vi "Format Page.vi"() -> ()   [LabVIEW 2020, in "3D Plot.lvclass"]
uses:
  <vilib>/Math Plots/3D Math Plots/3D Plot/3D Plot/3D Plot.lvclass
  <vilib>/Math Plots/3D Math Plots/3D Plot/3D Plot/Typedef/Format Property.ctl
  <vilib>/Math Plots/3D Math Plots/3D Plot/3D Plot/Typedef/Dialog State.ctl
  <vilib>/Math Plots/3D Math Plots/3D Plot/3D Plot/Typedef/Temp Scene State.ctl
  <vilib>/Math Plots/3D Math Plots/3D Plot/3D Plot/Typedef/Temp Scene Property Action.ctl
panel:
  out "Format Testing":string
  in  "Caption Texts":string[](array[string])=["Numeric Format Codes", "Absolute Time Format Codes\n(must be within %< >T)", "Relative Time Format Codes\n(must be within %< >t)"]
  in  "Item Names":string[][][](array[string])=[[["Floating point notation", "%f"], ["Scientific notation", "%e"], ["Engineering notation", "%^e"], ["Automatic notation", "%#_g"], ["SI notation", "%p"], ["Decimal", "%d"], ["Unsigned decimal", "%u"], ["Hexadecimal", "%x"], ["Octal", "%o"], ["Binary", "%b"], ["A single percent character", "%%"], ["", ""], ["", ""], ["", ""], ["", ""], ["", ""], ["", ""], ["", ""], ["", ""], ["", ""], ["", ""], ["", ""], ["", ""]], [["Absolute time container", "%< >T"], ["Abbreviated weekday name", "%a"], ["Weekday name", "%A"], ["Abbreviated month name", "%b"], ["Month name", "%B"], ["Default date and time", "%c"], ["Day of month (01-31)", "%d"], ["Hour (24-hour clock) (00-23)", "%H"], ["Hour (12-hour clock) (01-12)", "%I"], ["Day of year (001-366)", "%j"], ["Month number (01-12)", "%m"], ["Minute (00-59)", "%M"], ["AM or PM flag", "%p"], ["Seconds (00-59)", "%S"], ["Fractional seconds with <digit>\nprecision", "%<digit> u"], ["Week number (00-53) with\nSunday as the first day of week 1", "%U"], ["Weekday number (0-6)", "%w"], ["Week number (00-53) with\nMonday as the first day of week 1", "%W"], ["Locale date", "%x"], ["Locale time", "%X"], ["Year within century (00-99)", "%y"], ["Year including century", "%Y"], ["Time zone", "%Z"]], [["Relative time container", "%< >t"], ["Weeks", "%W"], ["Days", "%D"], ["Hours", "%H"], ["Minutes", "%M"], ["Seconds", "%S"], ["Fractional seconds with <digit>\nprecision", "%<digit>u"], ["A single percent character", "%%"], ["", ""], ["", ""], ["", ""], ["", ""], ["", ""], ["", ""], ["", ""], ["", ""], ["", ""], ["", ""], ["", ""], ["", ""], ["", ""], ["", ""], ["", ""]]]
  out "Advanced Tab":enum32{"Standard", "Advanced"}(tab)
  out "Time/Date Tab":enum32{"numeric", "time"}(tab) caption="Tab Control 3"
  in  "HLP_just/pad":i32(ring) items=["Pad with spaces on left", "Pad with spaces on right", "Pad with zeros on left"]
  in  "HLP_UseMinWidth":bool caption="Use minimum field width"
  in  "HLP_trailing zeros":bool caption="Hide trailing zeros"
  in  "HLP_exponent":bool caption="Exponent in multiples of 3"
  in  "Precision Type":u16(ring) caption="Precision type" items=["Digits of precision", "Significant digits"]
  in  "Digits":i32 min=0
  in  "HLP_Minimum field width":i32 caption="Minimum field width" min=0
  in  "HLP_year-new":T1(radio)
  in  "HLP_MDY 2-new":T1(radio)
  in  "HLP_HMS-new":enum32{"Radio Selection 1", "Radio Selection 2"}(radio)
  in  "HLP_Hour Type-new":enum32{"Radio Selection 1", "Radio Selection 2"}(radio)
  in  "HLP_Date Type":u16(ring)=1 caption="Date Type" items=["Custom date format", "System date format", "Date unused"]
  in  "HLP_Digits":i32 caption="Digits" min=0
  in  "HLP_Time Type":u16(ring)=1 caption="Time Type" items=["Custom time format", "System time format", "Time unused"]
  in  "Type":i32(listbox)
  in  "HLP_Revert":bool caption="Revert"
  in  "HLP_Format Code List Type":u16(ring) items=["Numeric format codes", "Relative time format codes", "Absolute time format codes"]
  out "HLP_Valid Fmt String":bool=TRUE caption="Valid"
  in  "HLP_insert format code":bool caption="Insert into Format String"
  in  "HLP_percent codes":i32(listbox) caption="Numeric Format Codes"
  in  "ODF_Format String":string caption="Format string"
  in  "HLP_AdvancedFmt2":enum32{"Default mode", "Advanced mode"}(radio)
  in  "Active Axis":u16(ring) caption="Active axis" items=["X Axis", "Y Axis", "Z Axis"]
  in  "Event Registration":refnum<event-registration>
  out "Format Property Out":T2
  in  "Format Property In":T2
  # "Format"
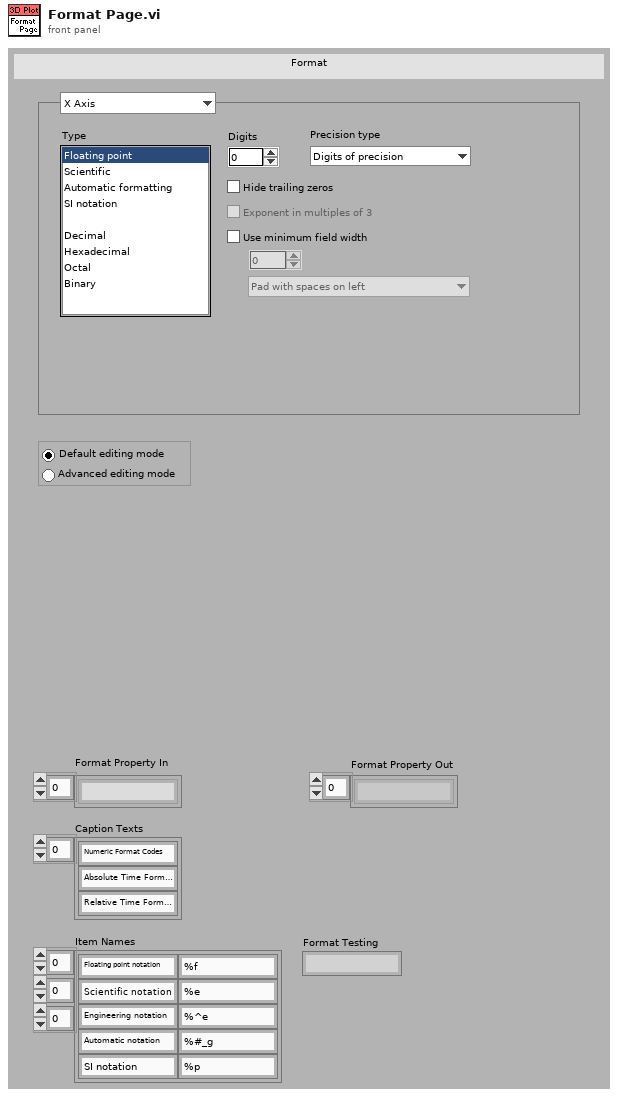
[diagram p1: front panel]
types:
  T1 = enum32{"Radio Selection 1", "Radio Selection 2", "Radio Selection 3"}
  T2 = typedef "3D Plot.lvclass/Format Property.ctl" = string[]
  T3 = typedef "3D Plot.lvclass/Dialog State.ctl" = enum16{"Initialize", "Read Porperty", "Write Property", "Idle", "Exit"}
  T4 = typedef "3D Plot.lvclass/Temp Scene Property Action.ctl" = enum16{"Graph Property", "Light Property", "Axis Property", "Value Pair Property", "Format Property", "Cursor Property", "Plot Specific Property"}
  T5 = typedef "3D Plot.lvclass/Temp Scene State.ctl" = enum16{"Create", "Update Scene", "Get Plot Representation", "Destory"}
  T6 = enum16{"number", "absolute time", "relative time"}
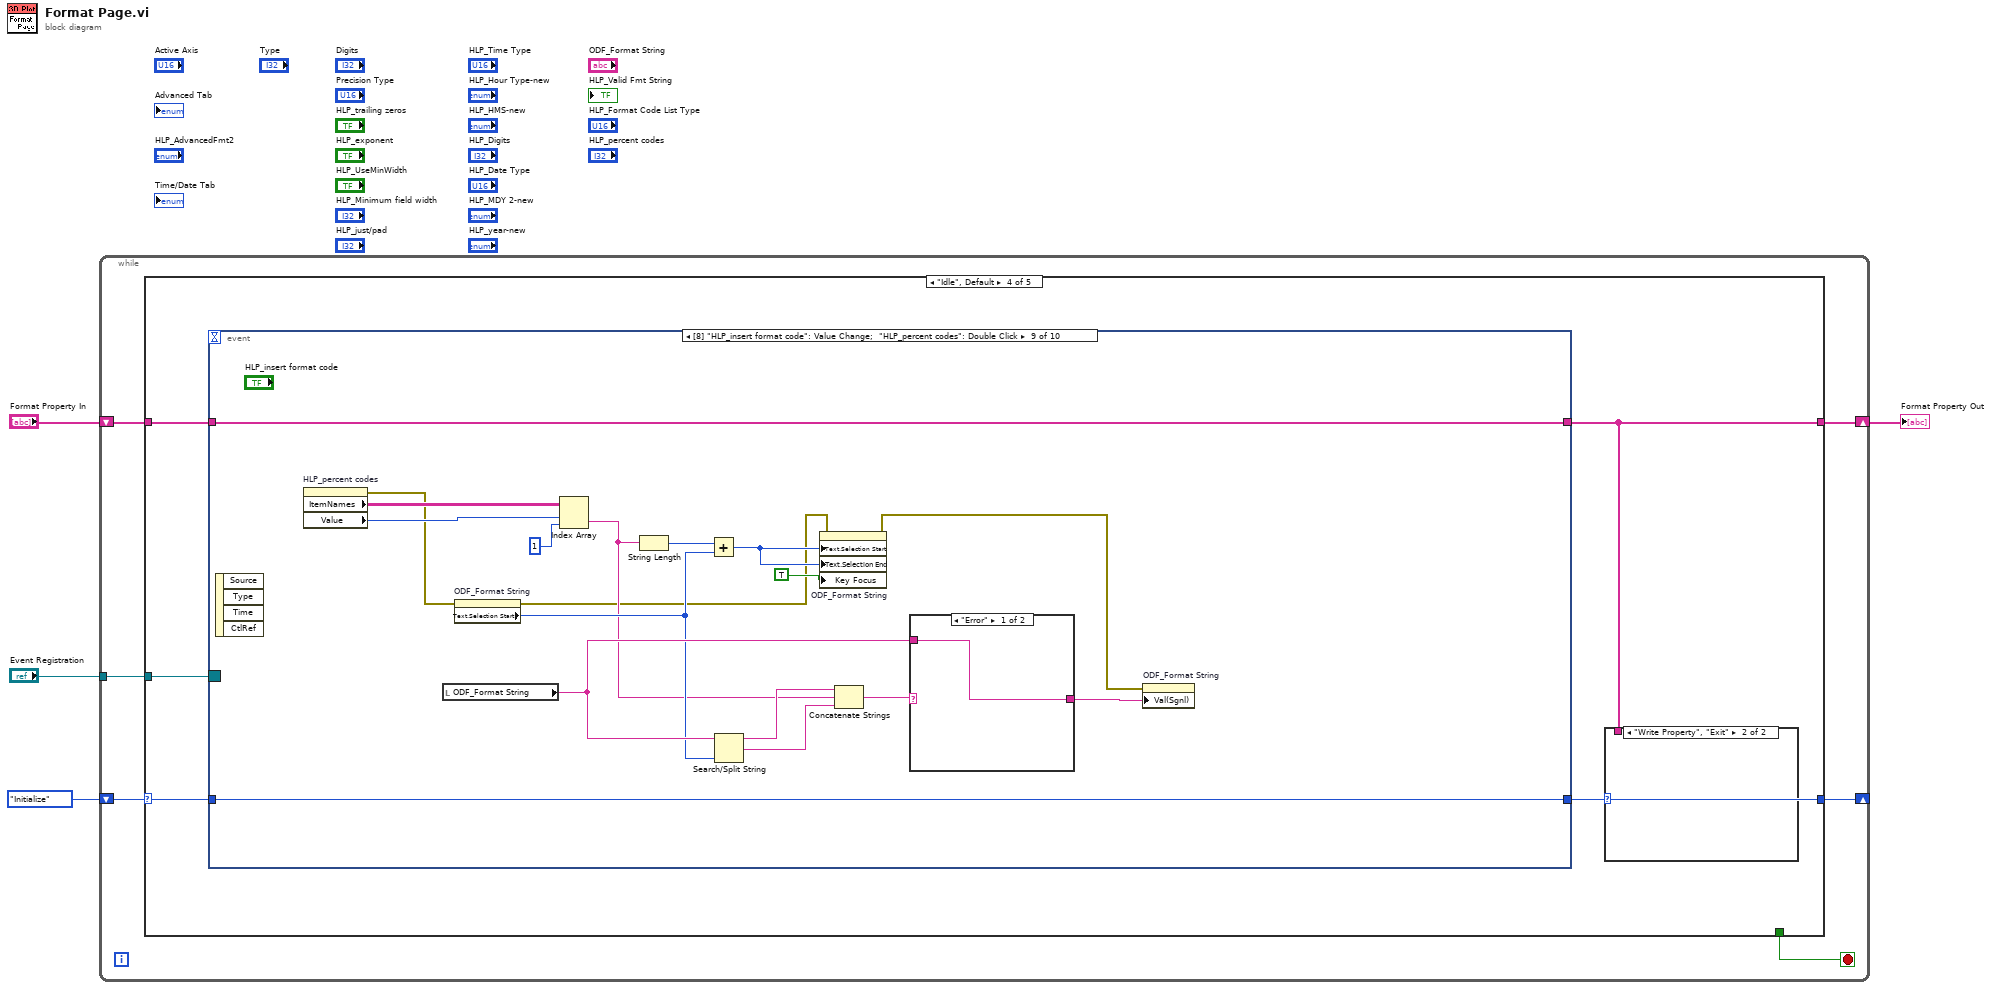
[diagram p0: block diagram]
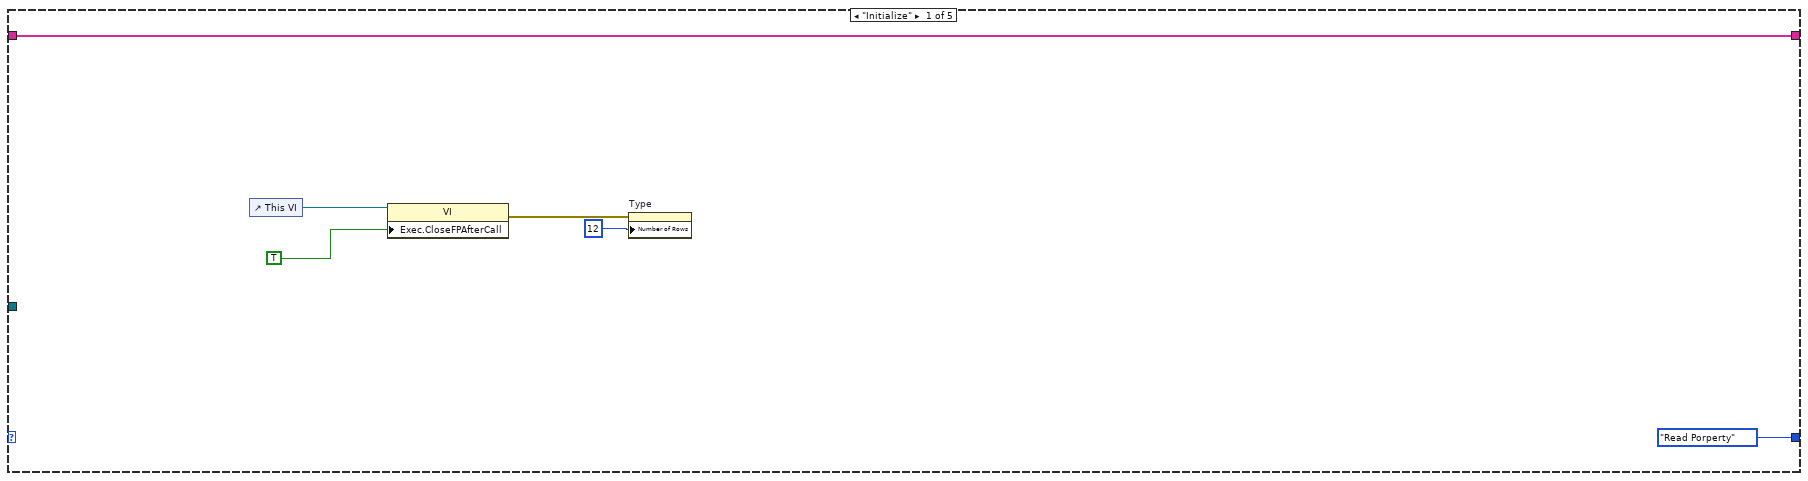
[diagram p2: hidden frame]
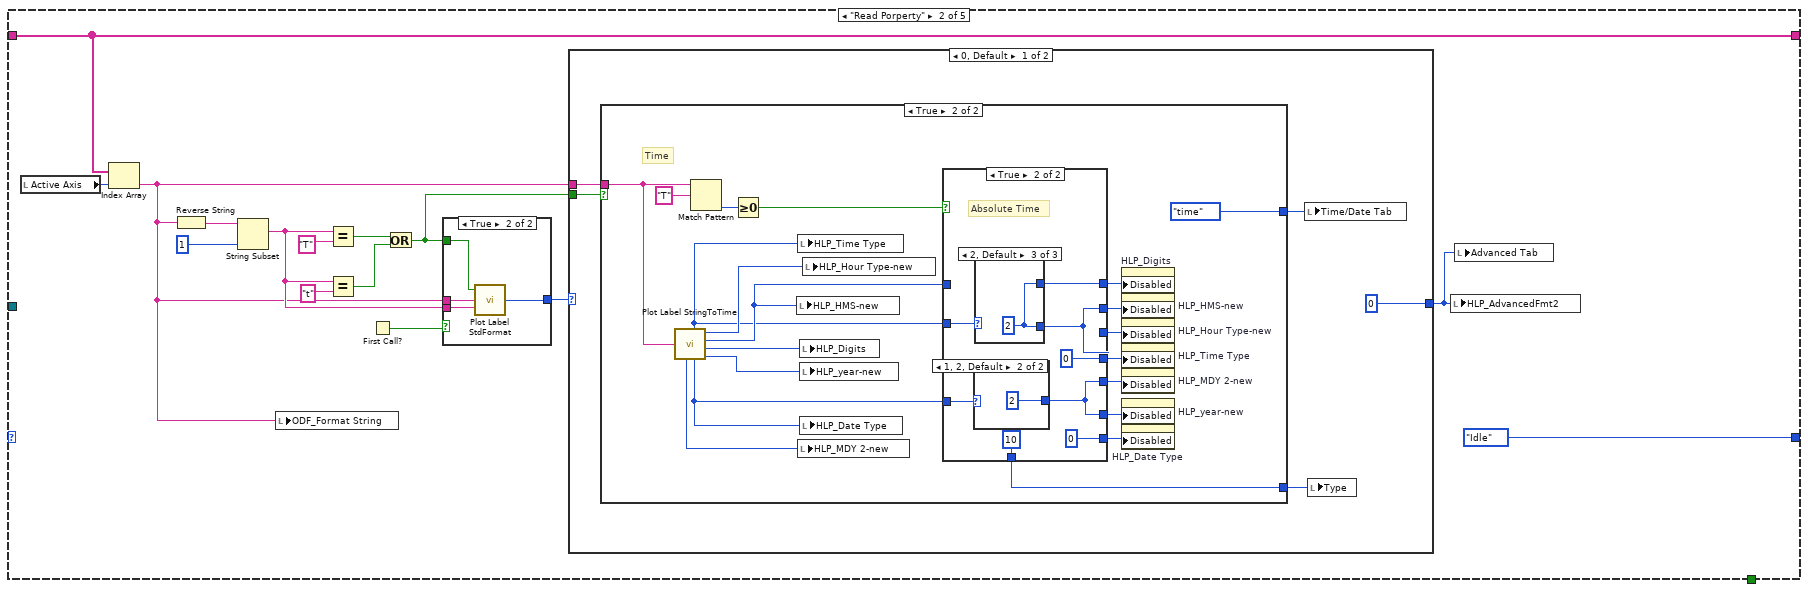
[diagram p3: hidden frame]
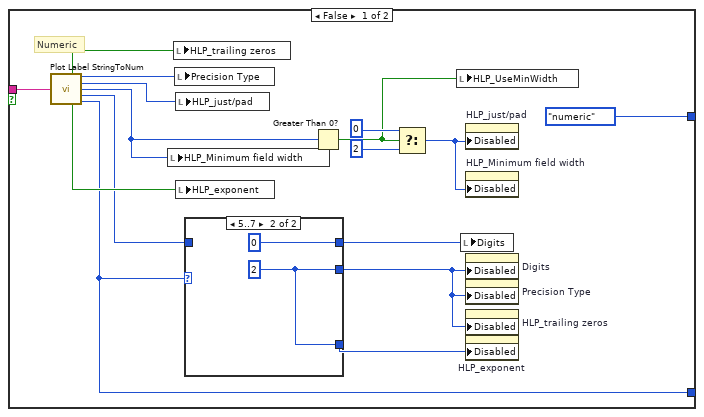
[diagram p4: hidden frame]
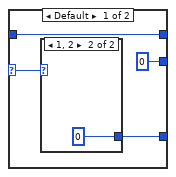
[diagram p5: hidden frame]
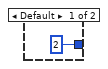
[diagram p6: hidden frame]
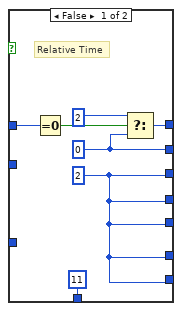
[diagram p7: hidden frame]
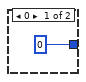
[diagram p8: hidden frame]
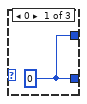
[diagram p9: hidden frame]
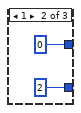
[diagram p10: hidden frame]
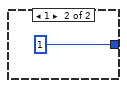
[diagram p11: hidden frame]
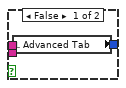
[diagram p12: hidden frame]
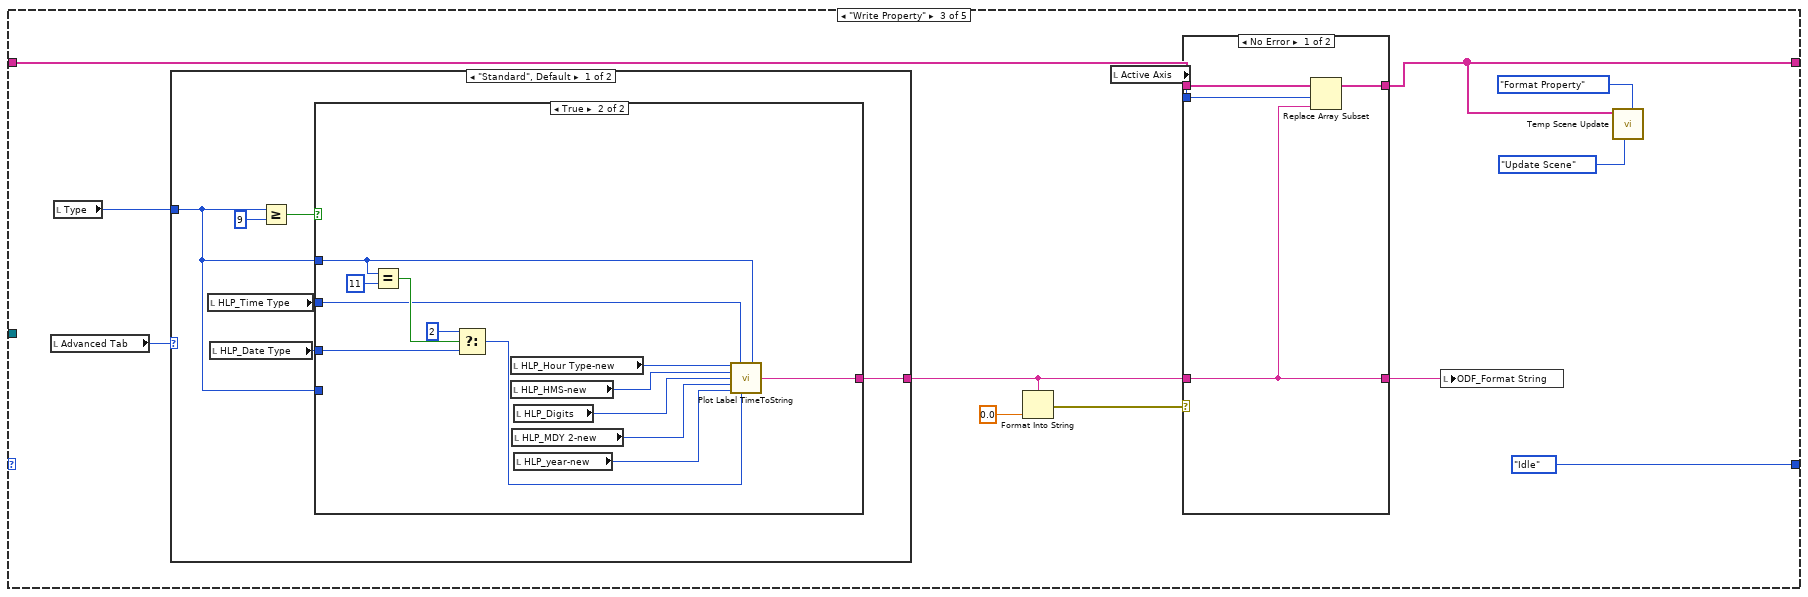
[diagram p13: hidden frame]
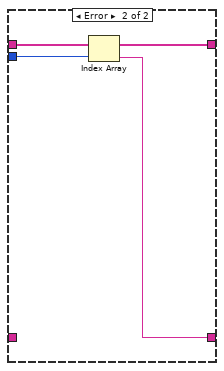
[diagram p14: hidden frame]
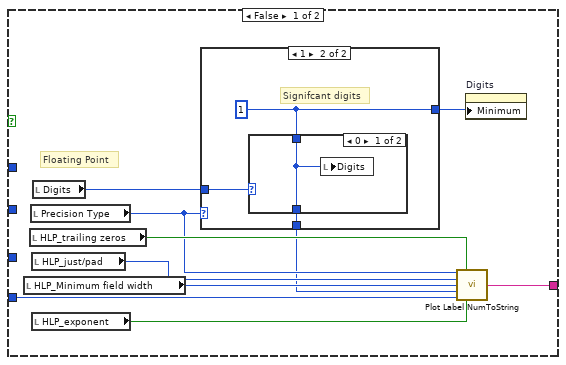
[diagram p15: hidden frame]
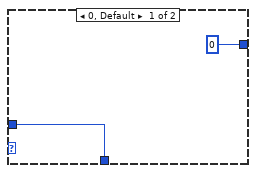
[diagram p16: hidden frame]
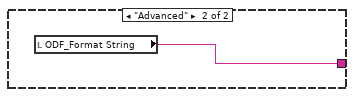
[diagram p18: hidden frame]
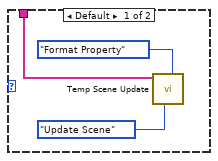
[diagram p19: hidden frame]
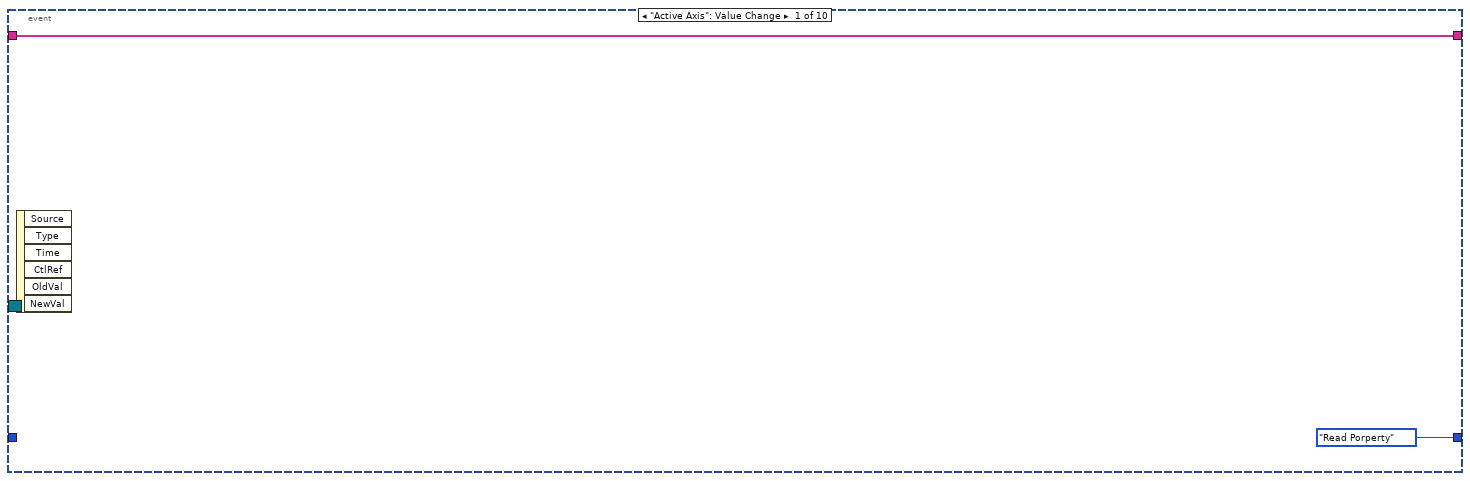
[diagram p20: hidden frame]
diagram:
  n1 = while {
    shift-right: [w5] -> w2
    shift-left: "Format Property In" -> [w10]
    shift-right: [w6] -> _
    shift-left: Dialog_State."Initialize" ("Enum") -> [w7]
    tunnel: "Event Registration" -> [w8]
    stop <- w9 stop-if-true
    n2 = case shown="\"Idle\", Default" w7 {
      selector: w7 -> [_ _ _ w166 _]
      tunnel: w10 -> [w16 w29 w114 w168 w387]
      tunnel: [w16 w29 w108 w165 w387] -> w5
      tunnel: [Dialog_State."Read Porperty" ("Enum") Dialog_State."Idle" Dialog_State."Idle" w164 Dialog_State."Exit"] -> w6
      tunnel: [_ _ _ _ TRUE] -> w9
      tunnel: w8 -> [_ _ _ w167 _]
      frame "Initialize" {
        n3 = control-ref of="This VI"() -> (w15:refnum<vi>)
        n4 = property class="VI"(reference=w15, "Exec.CloseFPAfterCall"=TRUE ("Execution:Close After Call")) -> (error out=w11:errorcluster)  [unwired: 1 in, 1 out]
        n5 = property on="Type" class="LstBox (strict)"(error in=w11, "Number of Rows"=u32 12) -> ()  [unwired: 1 in, 2 out]
      }
      frame "Read Porperty" {
        n6 = local read "Active Axis"() -> (w30:u16)
        n7 = Index Array(array=w29, index=w30) -> (element=w19:string)
        n8 = Reverse String(1:w19) -> (0:w24:string)
        n9 = String Subset(string=w24, length (rest)=1 ("length (rest)")) -> (substring=w28:string)  [unwired: 1 out]
        n10 = local write "ODF_Format String"(w19) -> ()
        n11 = Equal?(x=w28, y="T") -> (x = y?=w26:bool)
        n12 = Equal?(x=w28, y="t") -> (x = y?=w27:bool)
        n13 = First Call?() -> (First Call?: T/F=w21:bool)
        n14 = Or(x=w26, y=w27) -> (x .or. y?=w18:bool)
        n15 = case shown="True" w21 {
          tunnel: w28 -> [_ w105]
          tunnel: w18 -> [_ w107]
          tunnel: w19 -> [_ w106]
          tunnel: [w103 w104] -> w20
          frame False {
            n16 = local read "Advanced Tab"() -> (w103:enum32{"Standard", "Advanced"})
          }
          frame True {
            n17 = call <vilib>:"Plot Label StdFormat.vi"("Time Type"=w105, "Format String"=w106, "Type (false = numeric)"=w107) -> ("Custom"=w104:i32)
          }
        }
        n18 = case shown="0, Default" w20 {
          tunnel: w19 -> [w36 _]
          tunnel: w18 -> [w35 _]
          tunnel: [0 1] -> w17
          frame 0, Default {
            n19 = case shown="True" w35 {
              tunnel: w36 -> [w52 w78]
              tunnel: [w45 w69] -> w34
              tunnel: [enum32{"numeric", "time"}."numeric" ("Time/Date Tab") enum32{"numeric", "time"}."time" ("Time/Date Tab")] -> w33
              frame False {
                # "Numeric"
                n20 = call <vilib>:"Plot Label StringToNum.vi"("Format String"=w52) -> ("Hide trailing zeros"=w51:bool, "Digit Type"=w49:i32, "just/pad"=w48:i32, "Minimum Field Width"=w40:i32, "Digits of Precision"=w47:i32, "exponent"=w50:bool, "Numeric Format"=w45:i32)  [unwired: 8 out]
                n21 = local write "HLP_Minimum field width"(w40) -> ()
                n22 = local write "HLP_trailing zeros"(w51) -> ()
                n23 = local write "Precision Type"(w49) -> ()
                n24 = local write "HLP_just/pad"(w48) -> ()
                n25 = local write "HLP_exponent"(w50) -> ()
                n26 = case shown="5..7" w45 {
                  selector: w45 -> [w54 _]
                  tunnel: [u8 0 w59] -> w44
                  tunnel: w47 -> [w55 _]
                  tunnel: [w55 0 ("Digits of Precision")] -> w46
                  tunnel: [w53 w59] -> w43
                  frame Default {
                    n27 = case shown="1, 2" w54 {
                      tunnel: [u8 2 u8 0] -> w53
                      frame Default {
                      }
                      frame 1, 2 {
                      }
                    }
                  }
                  frame 5..7 {
                    w59 = u8 2
                  }
                }
                n28 = Greater Than 0?(x=w40) -> (x > 0?=w39:bool)
                n29 = Select(t=u8 0, s=w39, f=u8 2) -> (s? t:f=w38:u8)
                n30 = local write "HLP_UseMinWidth"(w39) -> ()
                n31 = local write "Digits"(w46) -> ()
                n32 = property on="HLP_just/pad" class="Ring (strict)"("Disabled"=w38) -> ()  [unwired: 2 in, 2 out]
                n33 = property on="HLP_Minimum field width" class="DigNum (strict)"("Disabled"=w38) -> ()  [unwired: 2 in, 2 out]
                n34 = property on="Digits" class="DigNum (strict)"("Disabled"=w44) -> ()  [unwired: 2 in, 2 out]
                n35 = property on="Precision Type" class="Ring (strict)"("Disabled"=w44) -> ()  [unwired: 2 in, 2 out]
                n36 = property on="HLP_trailing zeros" class="Bool (strict)"("Disabled"=w44) -> ()  [unwired: 2 in, 2 out]
                n37 = property on="HLP_exponent" class="Bool (strict)"("Disabled"=w43) -> ()  [unwired: 2 in, 2 out]
              }
              frame True {
                # "Time"
                n38 = call <vilib>:"Plot Label StringToTime.vi"("Time & Date Format String"=w78) -> ("MDY"=w76:i16, "Time Format"=w72:i16, "AM/PM"=w77:i16, "included seconds"=w73:i16, "Date Format"=w71:i16, "seconds precision"=w74:i16, "Year Format"=w75:i16)  [unwired: 3 out]
                n39 = Match Pattern(string=w78, regular expression="T") -> (offset past match=w80:i32)  [unwired: 4 out]
                n40 = Greater Or Equal To 0?(x=w80) -> (x >= 0?=w70:bool)
                n41 = local write "HLP_HMS-new"(w73) -> ()
                n42 = local write "HLP_Time Type"(w72) -> ()
                n43 = local write "HLP_MDY 2-new"(w76) -> ()
                n44 = local write "HLP_Digits"(w74) -> ()
                n45 = local write "HLP_year-new"(w75) -> ()
                n46 = local write "HLP_Date Type"(w71) -> ()
                n47 = local write "HLP_Hour Type-new"(w77) -> ()
                n48 = case shown="True" w70 {
                  tunnel: [w82 w95] -> w66
                  tunnel: [w87 w95] -> w65
                  tunnel: [w81 w88] -> w67
                  tunnel: [w87 0] -> w64
                  tunnel: [w87 0] -> w61
                  tunnel: [w87 w92] -> w62
                  tunnel: [w87 w92] -> w63
                  tunnel: w72 -> [_ w91]
                  tunnel: w71 -> [_ w90]
                  tunnel: [11 10] -> w69
                  tunnel: w73 -> [w83 _]
                  frame False {
                    w82 = 0
                    w87 = 2
                    # "Relative Time"
                    n49 = Equal To 0?(x=w83) -> (x = 0?=w84:bool)
                    n50 = Select(t=2, s=w84, f=w82) -> (s? t:f=w81:i32)
                  }
                  frame True {
                    # "Absolute Time"
                    n51 = case shown="1, 2, Default" w90 {
                      tunnel: [0 2] -> w92
                      frame 0 {
                      }
                      frame 1, 2, Default {
                      }
                    }
                    n52 = case shown="2, Default" w91 {
                      tunnel: [w98 2 w101] -> w95
                      tunnel: [w98 0 w101] -> w88
                      frame 0 {
                        w98 = 0
                      }
                      frame 1 {
                      }
                      frame 2, Default {
                        w101 = 2
                      }
                    }
                  }
                }
                n53 = property on="HLP_Digits" class="DigNum (strict)"("Disabled"=w67) -> ()  [unwired: 2 in, 2 out]
                n54 = property on="HLP_HMS-new" class="RadioBtnsControl (strict)"("Disabled"=w66) -> ()  [unwired: 2 in, 2 out]
                n55 = property on="HLP_Hour Type-new" class="RadioBtnsControl (strict)"("Disabled"=w65) -> ()  [unwired: 2 in, 2 out]
                n56 = property on="HLP_Time Type" class="Ring (strict)"("Disabled"=w64) -> ()  [unwired: 2 in, 2 out]
                n57 = property on="HLP_MDY 2-new" class="RadioBtnsControl (strict)"("Disabled"=w63) -> ()  [unwired: 2 in, 2 out]
                n58 = property on="HLP_year-new" class="RadioBtnsControl (strict)"("Disabled"=w62) -> ()  [unwired: 2 in, 2 out]
                n59 = property on="HLP_Date Type" class="Ring (strict)"("Disabled"=w61) -> ()  [unwired: 2 in, 2 out]
              }
            }
            n60 = local write "Time/Date Tab"(w33) -> ()
            n61 = local write "Type"(w34) -> ()
          }
          frame 1 {
          }
        }
        n62 = local write "HLP_AdvancedFmt2"(w17) -> ()
        n63 = local write "Advanced Tab"(w17) -> ()
      }
      frame "Write Property" {
        n64 = local read "Advanced Tab"() -> (w118:enum32{"Standard", "Advanced"})
        n65 = local read "Type"() -> (w117:i32)
        n66 = case shown="\"Standard\", Default" w118 {
          tunnel: w117 -> [w130 _]
          tunnel: [w127 w163] -> w113
          frame "Standard", Default {
            n67 = local read "HLP_Time Type"() -> (w129:u16)
            n68 = local read "HLP_Date Type"() -> (w128:u16)
            n69 = Greater Or Equal?(x=w130, y=9) -> (x >= y?=w131:bool)
            n70 = case shown="True" w131 {
              tunnel: w130 -> [_ w157]
              tunnel: w130 -> [w141 _]
              tunnel: w129 -> [_ w158]
              tunnel: w128 -> [_ w159]
              tunnel: [w142 w150] -> w127
              frame False {
                # "Floating Point"
                n71 = local read "HLP_Minimum field width"() -> (w139:i32)
                n72 = local read "HLP_trailing zeros"() -> (w138:bool)
                n73 = local read "Precision Type"() -> (w136:u16)
                n74 = local read "HLP_just/pad"() -> (w137:i32)
                n75 = local read "HLP_exponent"() -> (w140:bool)
                n76 = local read "Digits"() -> (w135:i32)
                n77 = case shown="1" w136 {
                  tunnel: w135 -> [w143 w147]
                  tunnel: [0 ("Data Range:Minimum") w146] -> w134
                  tunnel: [w143 w145] -> w133
                  frame 0, Default {
                  }
                  frame 1 {
                    w146 = 1 ("Data Range:Minimum")
                    # "Signifcant digits"
                    n78 = case shown="0" w147 {
                      selector: w147 -> [_ w149]
                      tunnel: w146 -> [w148 _]
                      tunnel: [w148 w149] -> w145
                      frame 0 {
                        n79 = local write "Digits"(w148) -> ()
                      }
                      frame 1, Default {
                      }
                    }
                  }
                }
                n80 = call <vilib>:"Plot Label NumToString.vi"("Digit Type"=w136, "Hide trailing zeros"=w138, "just/pad"=w137, "Minimum Field Width"=w139, "Digits of Precision"=w133, "Numeric Format"=w141, "exponent"=w140) -> ("Format String"=w142:string)  [unwired: 8 out]
                n81 = property on="Digits" class="DigNum (strict)"("Minimum"=w134) -> ()  [unwired: 2 in, 2 out]
              }
              frame True {
                n82 = Equal?(x=w157, y=11) -> (x = y?=w160:bool)
                n83 = Select(t=u16 2, s=w160, f=w159) -> (s? t:f=w151:u16)
                n84 = local read "HLP_Hour Type-new"() -> (w156:enum32{"Radio Selection 1", "Radio Selection 2"})
                n85 = local read "HLP_HMS-new"() -> (w155:enum32{"Radio Selection 1", "Radio Selection 2"})
                n86 = local read "HLP_MDY 2-new"() -> (w153:T1)
                n87 = local read "HLP_Digits"() -> (w154:i32)
                n88 = local read "HLP_year-new"() -> (w152:T1)
                n89 = call <vilib>:"Plot Label TimeToString.vi"("AM/PM"=w156, "Time Format"=w158, "Type (10 = Absolute)"=w157, "included seconds"=w155, "seconds precision"=w154, "m-d-y sequence"=w153, "year format"=w152, "Date Format"=w151) -> ("Format String"=w150:string)  [unwired: 3 in, 4 out]
              }
            }
          }
          frame "Advanced" {
            n90 = local read "ODF_Format String"() -> (w163:string)
          }
        }
        n91 = Format Into String(format string=w113, 0.0 ("input 1")) -> (error out=w115:errorcluster)  [unwired: 2 in, 1 out]
        n92 = local read "Active Axis"() -> (w112:u16)
        n93 = case shown="No Error" w115 {
          tunnel: w114 -> [w123 w124]
          tunnel: [w122 w124] -> w108
          tunnel: w113 -> [w120 _]
          tunnel: w112 -> [w121 w126]
          tunnel: [w120 w125] -> w111
          frame No Error {
            n94 = Replace Array Subset(array=w123, new element=w120, index=w121) -> (w122:T2)
          }
          frame Error {
            n95 = Index Array(array=w124, index=w126) -> (element=w125:string)
          }
        }
        n96 = local write "ODF_Format String"(w111) -> ()
        n97 = call <vilib>:"Temp Scene Update.vi"("Property Name"=Temp_Scene_Property_Action."Format Property", "State"=Temp_Scene_State."Update Scene", "Property In"=w108) -> ()  [unwired: 3 in, 6 out]
      }
      frame "Idle", Default {
        n98 = event shown="[8] \"HLP_insert format code\": Value Change;  \"HLP_percent codes\": Double Click" {
          selector: w167 -> [_ _ _ _ _ _ _ _ _ _]
          dyn-events: _ -> [_ _ _ _ _ _ _ _ _ _]
          timeout: _ -> [_ _ _ _ _ _ _ _ _ _]
          tunnel: w168 -> [w173 w174 w176 w247 w275 w280 w291 w359 w366 w386]
          tunnel: [w173 w174 w176 w246 w275 w280 w291 w359 w366 w386] -> w165
          tunnel: [Dialog_State."Read Porperty" Dialog_State."Write Property" Dialog_State."Write Property" w254 w276 Dialog_State."Write Property" w287 w358 w365 Dialog_State."Exit"] -> w164
          tunnel: w166 -> [_ _ _ w254 w276 _ w286 w358 w365 _]
          event "Active Axis": Value Change {
            n99 = event-data() -> ()  [unwired: 7 out]
          }
          event "HLP_Digits", "Digits", "HLP_just/pad", "HLP_exponent", "HLP_trailing zeros", "Precision Type", "HLP_Hour Type-new", "HLP_MDY 2-new", "HLP_year-new": Value Change {
            n100 = event-data() -> ()  [unwired: 7 out]
          }
          event "HLP_Date Type", "HLP_Time Type", "Type", "HLP_Minimum field width", "HLP_HMS-new": Value Change {
            n101 = event-data() -> ()  [unwired: 7 out]
            n102 = local read "HLP_AdvancedFmt2"() -> (w179:enum32{"Default mode", "Advanced mode"})
            n103 = local read "Type"() -> (w180:i32)
            n104 = case shown="\"Default mode\", Default" w179 {
              tunnel: w180 -> [w188 _]
              tunnel: [u32 0 u32 1] -> w178
              frame "Default mode", Default {
                n105 = case shown="Default" w188 {
                  selector: w188 -> [w237 _]
                  tunnel: [u8 0 w242] -> w197
                  tunnel: [w238 w242] -> w198
                  frame Default {
                    n106 = case shown="Default" w237 {
                      tunnel: [u8 2 u8 0] -> w238
                      frame Default {
                      }
                      frame 1, 2 {
                      }
                    }
                  }
                  frame 5..8 {
                    w242 = u8 2
                  }
                }
                n107 = Greater Or Equal?(x=w188, y=9) -> (x >= y?=w200:bool)
                n108 = Equal?(x=w188, y=11) -> (x = y?=w189:bool)
                n109 = Boolean To (0,1)(Boolean=w200) -> (0, 1=w199:i16)
                n110 = local write "Time/Date Tab"(w199) -> ()
                n111 = property on="HLP_exponent" class="Bool (strict)"("Disabled"=w198) -> ()  [unwired: 2 in, 2 out]
                n112 = property on="Precision Type" class="Ring (strict)"("Disabled"=w197) -> ()  [unwired: 2 in, 2 out]
                n113 = property on="HLP_trailing zeros" class="Bool (strict)"("Disabled"=w197) -> ()  [unwired: 2 in, 2 out]
                n114 = property on="Digits" class="DigNum (strict)"("Disabled"=w197) -> ()  [unwired: 2 in, 2 out]
                n115 = local read "HLP_Minimum field width"() -> (w194:i32)
                n116 = case shown="False" w189 {
                  tunnel: [w207 w233] -> w187
                  tunnel: [w206 w232] -> w186
                  tunnel: [w202 w231] -> w185
                  tunnel: [w205 w231] -> w184
                  tunnel: [w204 w231] -> w183
                  tunnel: [w203 w231] -> w182
                  tunnel: [w202 w231] -> w181
                  frame False {
                    w202 = u8 0
                    # "Absolute Time"
                    n117 = local read "HLP_Time Type"() -> (w209:u16)
                    n118 = local read "HLP_Date Type"() -> (w208:u16)
                    n119 = call <vilib>:"Plot subChangeDetector.vi"("value"=w209) -> ("changed?"=w210:bool)  [unwired: 10 out]
                    n120 = Equal?(x=2, y=w209) -> (x = y?=w213:bool)
                    n121 = Equal?(x=2, y=w208) -> (x = y?=w212:bool)
                    n122 = And(x=w213, y=w212) -> (x .and. y?=w211:bool)
                    n123 = case shown="True" w211 {
                      tunnel: w210 -> [_ w228]
                      tunnel: w209 -> [w220 _]
                      tunnel: w208 -> [w219 _]
                      tunnel: [w218 w227] -> w207
                      tunnel: [w217 w227] -> w206
                      tunnel: [w217 w227] -> w205
                      tunnel: [w216 w227] -> w204
                      tunnel: [w216 w227] -> w203
                      frame False {
                        n124 = case shown="2, Default" w220 {
                          tunnel: [w223 u8 2 w226] -> w217
                          tunnel: [w223 u8 0 w226] -> w218
                          frame 0 {
                            w223 = u8 0
                          }
                          frame 1 {
                          }
                          frame 2, Default {
                            w226 = u8 2
                          }
                        }
                        n125 = case shown="1, 2, Default" w219 {
                          tunnel: [u8 0 u8 2] -> w216
                          frame 0 {
                          }
                          frame 1, 2, Default {
                          }
                        }
                      }
                      frame True {
                        w227 = u8 2
                        n126 = case shown="False" w228 {
                          frame False {
                            w229 = u16 1 items=["Custom Date Format", "System Date Format", "Date Unused"] ("Date Type")
                            n127 = local write "HLP_Date Type"(w229) -> ()
                          }
                          frame True {
                            w230 = u16 1 items=["Custom Time Format", "System Time Format", "Time Unused"] ("Time Type")
                            n128 = local write "HLP_Time Type"(w230) -> ()
                          }
                        }
                      }
                    }
                  }
                  frame True {
                    w231 = u8 2
                    w232 = u8 0
                    # "Relative Time"
                    n129 = local read "HLP_HMS-new"() -> (w234:enum32{"Radio Selection 1", "Radio Selection 2"})
                    n130 = Equal To 0?(x=w234) -> (x = 0?=w236:bool)
                    n131 = Select(t=u8 2, s=w236, f=w232) -> (s? t:f=w233:u8)
                  }
                }
                n132 = Greater Than 0?(x=w194) -> (x > 0?=w193:bool)
                n133 = Select(t=u8 0, s=w193, f=u8 2) -> (s? t:f=w192:u8)
                n134 = local write "HLP_UseMinWidth"(w193) -> ()
                n135 = property on="HLP_Minimum field width" class="DigNum (strict)"("Disabled"=w192) -> ()  [unwired: 2 in, 2 out]
                n136 = property on="HLP_just/pad" class="Ring (strict)"("Disabled"=w192) -> ()  [unwired: 2 in, 2 out]
                n137 = property on="HLP_Digits" class="DigNum (strict)"("Disabled"=w187) -> ()  [unwired: 2 in, 2 out]
                n138 = property on="HLP_HMS-new" class="RadioBtnsControl (strict)"("Disabled"=w186) -> ()  [unwired: 2 in, 2 out]
                n139 = property on="HLP_Hour Type-new" class="RadioBtnsControl (strict)"("Disabled"=w184) -> ()  [unwired: 2 in, 2 out]
                n140 = property on="HLP_Time Type" class="Ring (strict)"("Disabled"=w185) -> ()  [unwired: 2 in, 2 out]
                n141 = property on="HLP_MDY 2-new" class="RadioBtnsControl (strict)"("Disabled"=w183) -> ()  [unwired: 2 in, 2 out]
                n142 = property on="HLP_year-new" class="RadioBtnsControl (strict)"("Disabled"=w182) -> ()  [unwired: 2 in, 2 out]
                n143 = property on="HLP_Date Type" class="Ring (strict)"("Disabled"=w181) -> ()  [unwired: 2 in, 2 out]
              }
              frame "Advanced mode" {
              }
            }
            n144 = local write "Advanced Tab"(w178) -> ()
          }
          event "ODF_Format String": Value Change {
            n145 = event-data() -> ("NewVal"=w245:string)  [unwired: 1 out]
            n146 = Format Into String(format string=w245, 0.0 ("input 1")) -> (resulting string=→"Format Testing":string, error out=w248:errorcluster)  [unwired: 2 in]
            n147 = local read "HLP_Valid Fmt String"() -> (w251:bool)
            n148 = Unbundle By Name(w248) -> ("status"=w250:bool)
            n149 = Not(x=w251) -> (.not. x?=w252:bool)
            n150 = And(x=w252, y=w250) -> (x .and. y?=w249:bool)
            n151 = case shown="False" w249 {
              tunnel: w248 -> [w260 _]
              tunnel: w247 -> [w257 w270]
              tunnel: [w256 w270] -> w246
              tunnel: w245 -> [w255 _]
              frame False {
                n152 = case shown="Error" w260 {
                  tunnel: [TRUE FALSE] -> w259
                  tunnel: [u8 2 u8 0] -> w258
                  tunnel: w257 -> [w264 w267]
                  tunnel: [w263 w267] -> w256
                  tunnel: w255 -> [w262 _]
                  frame No Error {
                    n153 = local read "Active Axis"() -> (w261:u16)
                    n154 = Replace Array Subset(array=w264, new element=w262, index=w261) -> (w263:T2)
                  }
                  frame Error {
                  }
                }
                n155 = local write "HLP_Valid Fmt String"(w259) -> ()
                n156 = property on="HLP_Revert" class="Bool"("Disabled"=w258) -> ()  [unwired: 2 in, 2 out]
              }
              frame True {
              }
            }
          }
          event "HLP_Revert": Value Change {
            n157 = event-data() -> ()  [unwired: 7 out]
            n158 = local read "Active Axis"() -> (w274:u16)
            n159 = Index Array(array=w275, index=w274) -> (element=w273:string)
            n160 = local write "HLP_Valid Fmt String"(TRUE ("HLP_Valid Fmt String")) -> ()
            n161 = local write "ODF_Format String"(w273) -> ()
            n162 = property on="HLP_Revert" class="Bool"("Disabled"=u8 2) -> ()  [unwired: 2 in, 2 out]
          }
          event "HLP_UseMinWidth": Value Change {
            n163 = event-data() -> ("NewVal"=w279:bool)  [unwired: 1 out]
            n164 = case shown="True" w279 {
              tunnel: [u8 2 u8 0] -> w278
              tunnel: [0 1] -> w277
              frame False {
              }
              frame True {
              }
            }
            n165 = local write "HLP_Minimum field width"(w277) -> ()
            n166 = property on="HLP_just/pad" class="Ring (strict)"("Disabled"=w278) -> ()  [unwired: 2 in, 2 out]
            n167 = property on="HLP_Minimum field width" class="DigNum (strict)"("Disabled"=w278) -> ()  [unwired: 2 in, 2 out]
          }
          event "HLP_AdvancedFmt2": Value Change {
            # "Reset these booleans Reset when changing to either tab because when going to advanced, you can't have a bad format string.  When going to simple mode, we reset these because we coerce to a good format string."
            n168 = event-data() -> ("NewVal"=w292:enum32{"Default mode", "Advanced mode"})  [unwired: 1 out]
            n169 = case shown="\"Default mode\", Default" w292 {
              tunnel: w291 -> [w309 _]
              tunnel: [0 1] -> w290
              tunnel: [TRUE ("HLP_Valid Fmt String") TRUE ("HLP_Valid Fmt String")] -> w288
              tunnel: [Dialog_State."Read Porperty" ("Enum") w346] -> w287
              tunnel: w286 -> [_ w346]
              frame "Default mode", Default {
                # "Switching from simple to advanced editing mode.\nThis case determines if the current format string can be represented by the basic selection controls.  If not, the format string is coerced to something that can be represented by the simple controls.  When coerced, the format string property is written, to update the control.  Whether coerced or not, the next event is Read Properties so that the controls are set up properly in the UI.\n\nIf the current format string in advanced was good, we use it.  If not, we use the last known good format string.  So, switching back to simple mode is a way for users to get out of a bad format string situation."
                n170 = local read "Active Axis"() -> (w308:u16)
                n171 = local read "ODF_Format String"() -> (w295:string)
                n172 = local read "HLP_Valid Fmt String"() -> (w307:bool)
                n173 = Index Array(array=w309, index=w308) -> (element=w306:string)
                n174 = Select(t=w295, s=w307, f=w306) -> (s? t:f=w298:string)
                n175 = Reverse String(1:w298) -> (0:w305:string)
                n176 = String Subset(string=w305, length (rest)=1 ("length (rest)")) -> (substring=w297:string)  [unwired: 1 out]
                n177 = Equal?(x=w297, y="T") -> (x = y?=w302:bool)
                n178 = Equal?(x=w297, y="t") -> (x = y?=w303:bool)
                n179 = Or(x=w302, y=w303) -> (x .or. y?=w299:bool)
                n180 = case shown="False" w299 {
                  tunnel: w298 -> [w311 w343]
                  tunnel: w297 -> [_ w342]
                  tunnel: [w312 w340] -> w296
                  frame False {
                    n181 = call <vilib>:"Plot Label StdFormat.vi"("Format String"=w311) -> ("Custom"=w313:i32)  [unwired: 2 in]
                    n182 = case shown="1" w313 {
                      tunnel: [w314 w315] -> w312
                      tunnel: w311 -> [w314 w323]
                      frame 0, Default {
                        # "Not a custom value.  Keep\nformat"
                      }
                      frame 1 {
                        # "Custom format.  Coerce.\nNote, ideally the page should not\ncoerce unless the user changes format\nin the default page."
                        n183 = call <vilib>:"Plot Label StringToNum.vi"("Format String"=w323) -> ("Hide trailing zeros"=w316:bool, "Digit Type"=w321:i32, "just/pad"=w320:i32, "Minimum Field Width"=w319:i32, "Digits of Precision"=w318:i32, "exponent"=w317:bool, "Numeric Format"=w322:i32)  [unwired: 8 out]
                        n184 = case shown="Default" w322 {
                          tunnel: w322 -> [_ w332]
                          tunnel: w321 -> [_ w331]
                          tunnel: w320 -> [_ w330]
                          tunnel: w319 -> [_ w329]
                          tunnel: w318 -> [_ w328]
                          tunnel: w317 -> [_ w327]
                          tunnel: w316 -> [_ w326]
                          tunnel: ["%.0f" w325] -> w315
                          frame -1 {
                          }
                          frame Default {
                            n185 = call <vilib>:"Plot Label NumToString.vi"("Digit Type"=w331, "Hide trailing zeros"=w326, "just/pad"=w330, "Minimum Field Width"=w329, "Digits of Precision"=w328, "Numeric Format"=w332, "exponent"=w327) -> ("Format String"=w325:string)  [unwired: 8 out]
                          }
                        }
                      }
                    }
                  }
                  frame True {
                    n186 = call <vilib>:"Plot Label StringToTime.vi"("Time & Date Format String"=w343) -> ("MDY"=w334:i16, "Time Format"=w339:i16, "AM/PM"=w338:i16, "included seconds"=w337:i16, "Date Format"=w333:i16, "seconds precision"=w336:i16, "Year Format"=w335:i16)  [unwired: 3 out]
                    n187 = case shown="\"t\"" w342 {
                      tunnel: [10 11] -> w341
                      frame "T", Default {
                      }
                      frame "t" {
                      }
                    }
                    n188 = call <vilib>:"Plot Label TimeToString.vi"("AM/PM"=w338, "Time Format"=w339, "Type (10 = Absolute)"=w341, "included seconds"=w337, "seconds precision"=w336, "m-d-y sequence"=w334, "year format"=w335, "Date Format"=w333) -> ("Format String"=w340:string)  [unwired: 3 in, 4 out]
                  }
                }
                n189 = local write "ODF_Format String"(w296) -> ()
              }
              frame "Advanced mode" {
                # "Switching from advanced to simple editing mode.\nThis case sets up the correct advanced format string table based on format type.  \n\nDon't go to read or write properties because the advanced tab shows the format string and it should be kept up-to-date by other events."
                n190 = local read "Type"() -> (w354:i32)
                n191 = case shown="9" w354 {
                  tunnel: [T6."number" ("Enum") T6."absolute time" ("Enum") T6."relative time" ("Enum")] -> w353
                  frame 0, Default {
                  }
                  frame 9 {
                  }
                  frame 10 {
                  }
                }
                n192 = Index Array(array="Item Names", index (dim 0)=w353) -> (element=w349:string[][])  [unwired: 2 in]
                n193 = Index Array(array="Caption Texts", index=w353) -> (element=w350:string)
                n194 = property on="HLP_percent codes" class="MCListbox (strict)"("ItemNames"=w349, "Caption.Text"=w350) -> ()  [unwired: 2 in, 2 out]
              }
            }
            n195 = local write "HLP_Valid Fmt String"(w288) -> ()
            n196 = local write "Advanced Tab"(w290) -> ()
            n197 = property on="HLP_Revert" class="Bool"("Disabled"=u8 2) -> ()  [unwired: 2 in, 2 out]
          }
          event "HLP_Format Code List Type": Value Change {
            n198 = event-data() -> ("NewVal"=w360:u16)  [unwired: 1 out]
            n199 = local read "Item Names"() -> (w362:string[][][])
            n200 = local read "Caption Texts"() -> (w361:string[])
            n201 = Index Array(array=w362, index (dim 0)=w360) -> (element=w363:string[][])  [unwired: 2 in]
            n202 = Index Array(array=w361, index=w360) -> (element=w364:string)
            n203 = property on="HLP_percent codes" class="MCListbox (strict)"("ItemNames"=w363, "Caption.Text"=w364) -> ()  [unwired: 2 in, 2 out]
          }
          event "HLP_insert format code": Value Change; "HLP_percent codes": Double Click {
            n204 = event-data() -> ()  [unwired: 5 out]
            n205 = property on="HLP_percent codes" class="MCListbox (strict)"() -> (error out=w367:errorcluster, "ItemNames"=w382:string[][], "Value"=w380:i32)  [unwired: 2 in, 1 out]
            n206 = local read "ODF_Format String"() -> (w374:string)
            n207 = property on="ODF_Format String" class="Str"(error in=w367) -> (error out=w369:errorcluster, "Text.Selection Start"=w372:u32)  [unwired: 1 in, 1 out]
            n208 = Index Array(array=w382, index (row)=w380, index (col)=1 ("disabled index (col)")) -> (element=w371:string)
            n209 = String Length(string=w371) -> (length=w379:i32)
            n210 = Add(x=w379, y=w372) -> (x+y=w378:u32)
            n211 = Search/Split String(string=w374, offset (0)=w372) -> (substring before match=w376:string, match + rest of string=w375:string)  [unwired: 2 out]
            n212 = property on="ODF_Format String" class="Str"(error in=w369, "Text.Selection Start"=w378, "Text.Selection End"=w378, "Key Focus"=TRUE) -> (error out=w368:errorcluster)  [unwired: 1 in, 1 out]
            n213 = Concatenate Strings(w376, w371, w375) -> (w373:string)
            n214 = case shown="\"Error\"" w373 {
              selector: w373 -> [_ w384]
              tunnel: w374 -> [w383 _]
              tunnel: [w383 w384] -> w370
              frame "Error" {
              }
              frame "No Error", Default {
              }
            }
            n215 = property on="ODF_Format String" class="Str"(error in=w368, "Val(Sgnl)"=w370) -> ()  [unwired: 1 in, 2 out]
          }
          event User Event {
            n216 = event-data() -> ()  [unwired: 6 out]
          }
        }
        n217 = case shown="\"Write Property\", \"Exit\"" w164 {
          tunnel: w165 -> [w169 _]
          frame Default {
            n218 = call <vilib>:"Temp Scene Update.vi"("Property Name"=Temp_Scene_Property_Action."Format Property", "State"=Temp_Scene_State."Update Scene", "Property In"=w169) -> ()  [unwired: 3 in, 6 out]
          }
          frame "Write Property", "Exit" {
          }
        }
      }
      frame "Exit" {
      }
    }
  }
  "Format Property Out" <- w2
